vi "Parametrize.vi"(11 "Raw Data":dbl[][](array[numeric])) -> (3 "Poperties":T1)   [LabVIEW 2019]
uses:
  Communication/TypeDef/#TypeDef_PropertiesToSave.ctl
  Global_Freq.vi
  <vilib>/Analysis/NI_AALBase.lvlib
  <vilib>/Analysis/baseanly.llb/Mean (DBL).vi
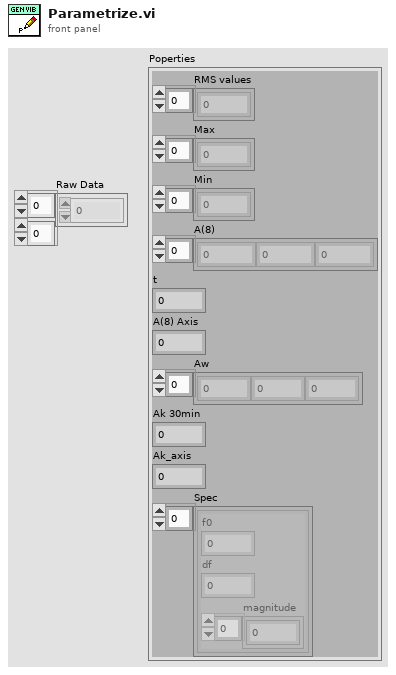
[diagram p1: front panel]
types:
  T1 = typedef "#TypeDef_PropertiesToSave.ctl" = cluster{"RMS values":dbl[], "Max":dbl[], "Min":dbl[], "A(8)":dbl[], "t":dbl, "A(8) Axis":dbl, "Aw":dbl[], "Ak 30min":dbl, "Ak_axis":i32, "Spec":cluster{"f0":dbl, "df":dbl, "magnitude":dbl[]}[]}
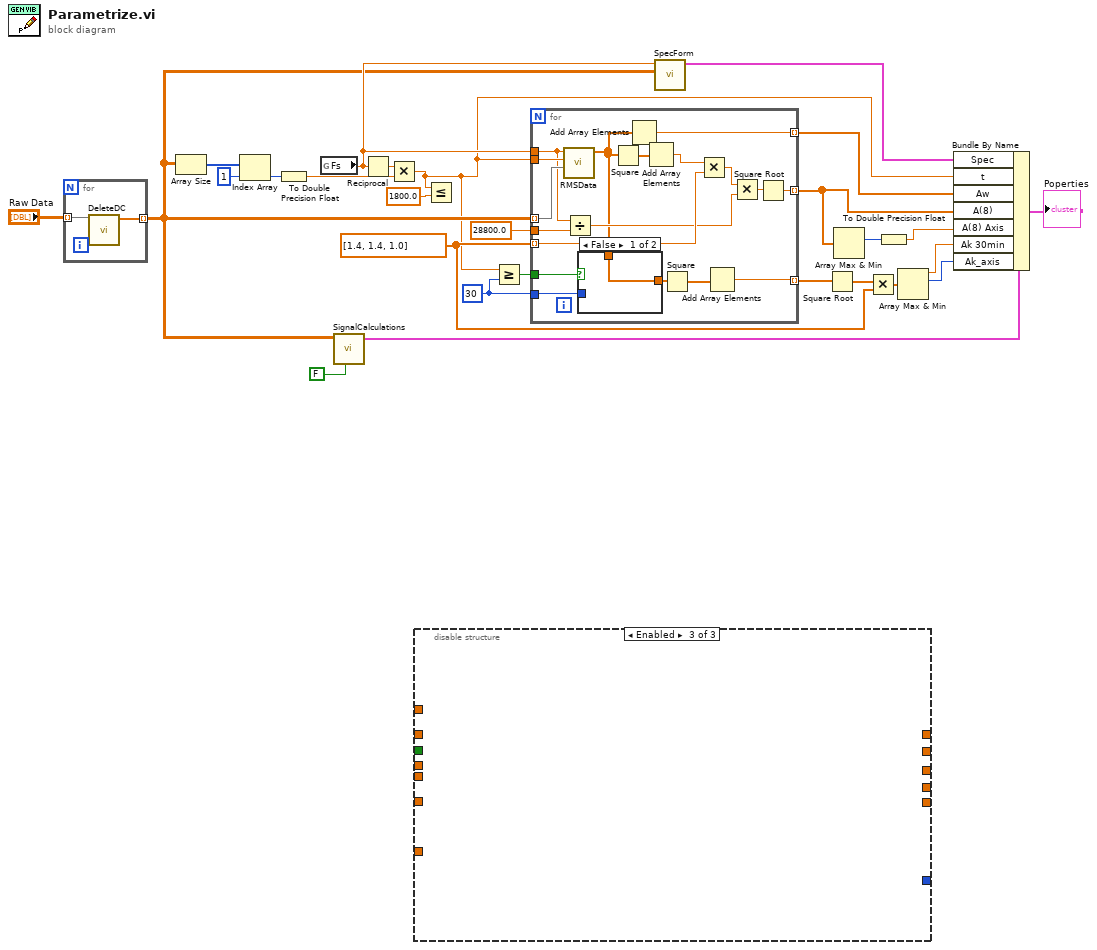
[diagram p0: block diagram]
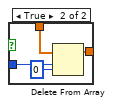
[diagram p2: hidden frame]
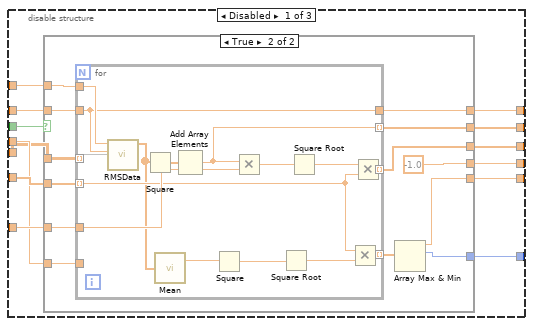
[diagram p3: hidden frame]
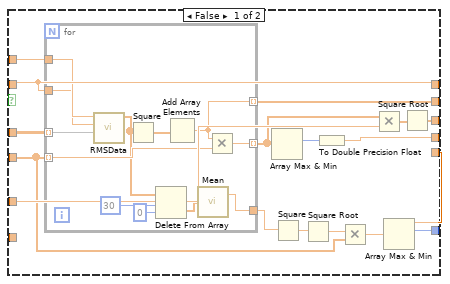
[diagram p4: hidden frame]
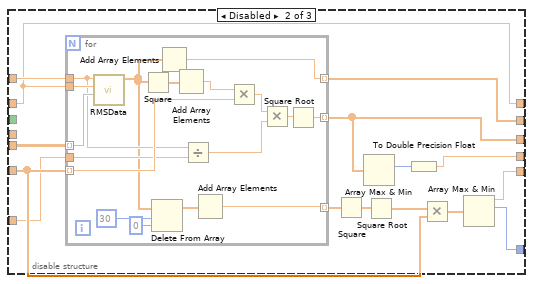
[diagram p5: hidden frame]
diagram:
  w3 = 30 ("length")
  w17 = dbl[] [1.4, 1.4, 1.0]
  n1 = for {
    tunnel: "Raw Data" -> [w29] mode=indexing
    tunnel: [w28] -> w8 mode=indexing
    n2 = call "DeleteDC.vi"("element"=w29) -> ("Array"=w28:dbl[])  [unwired: 10 in]
  }
  n3 = Array Size(array=w8) -> (size(s)=w18:i32[])
  n4 = Index Array(array=w18, index=1) -> (element=w20:i32)
  n5 = To Double Precision Float(number=w20) -> (double precision float=w14:dbl)
  n6 = global read "Global_Freq.vi" "Fs"() -> (w10:dbl)
  n7 = call "SignalCalculations.vi"("Ref?"=FALSE, "All Data"=w8) -> ("Poperties"=w23:T1)  [unwired: 8 in, 1 out]
  n8 = Reciprocal(x=w10) -> (1/x=w21:dbl)
  n9 = Multiply(x=w21, y=w14) -> (x*y=w2:dbl)
  n10 = disable-structure shown="Enabled" {
    disable-tunnel: [w42 w103 _] -> _
    disable-tunnel: [w41 w100 _] -> _
    disable-tunnel: [w40 w102 _] -> _
    disable-tunnel: [w39 w111 _] -> _
    disable-tunnel: _ -> [w38 w101 _]
    disable-tunnel: _ -> [w37 _ _]
    disable-tunnel: _ -> [w36 w111 _]
    disable-tunnel: _ -> [w35 w106 _]
    disable-tunnel: [w34 w105 _] -> _
    disable-tunnel: [w33 w104 _] -> _
    disable-tunnel: _ -> [w32 _ _]
    disable-tunnel: _ -> [w31 w112 _]
    disable-tunnel: _ -> [w30 w114 _]
    frame Disabled {
      n11 = case shown="True" w37 {
        tunnel: w35 -> [w43 w84]
        tunnel: [w57 w83] -> w41
        tunnel: w30 -> [w54 w82]
        tunnel: w36 -> [w44 w81]
        tunnel: w38 -> [w59 w80]
        tunnel: [w50 w79] -> w40
        tunnel: [w44 w78] -> w39
        tunnel: [w55 -1.0] -> w42
        tunnel: w32 -> [_ w76]
        tunnel: [w51 w74] -> w34
        tunnel: [w49 w73] -> w33
        tunnel: w31 -> [w45 w72]
        frame False {
          n12 = for {
            tunnel: w43 -> [w71] mode=indexing
            tunnel: w54 -> [w68] mode=indexing
            tunnel: [w70] -> w46 mode=indexing
            tunnel: [w66] -> w50 mode=indexing
            tunnel: [w60] -> w48
            tunnel: w45 -> [w64]
            tunnel: w44 -> [w63]
            n13 = call "RMSData.vi"("Data in"=w68, "t"=w63, "Fs"=w64) -> ("RMS Data out"=w62:dbl[])  [unwired: 8 in]
            n14 = Square(x=w62) -> (x^2=w67:dbl[])
            n15 = Delete From Array(array=w62, length=30, index=0) -> (deleted portion=w61:dbl[])  [unwired: 1 out]
            n16 = Add Array Elements(numeric array=w67) -> (sum=w66:dbl)
            n17 = call-poly <vilib>:"Mean.vi"("X"=w61) -> ("mean"=w60:dbl)  [unwired: 1 out]
            n18 = Multiply(x=w66, y=w71) -> (x*y=w70:dbl)
          }
          n19 = Array Max & Min(array=w46) -> (max index (indices)=w56:i32)  [unwired: 3 out]
          n20 = Square(x=w48) -> (x^2=w47:dbl)
          n21 = Square Root(x=w47) -> (sqrt(x)=w53:dbl)
          n22 = To Double Precision Float(number=w56) -> (double precision float=w55:dbl)
          n23 = Multiply(x=w53, y=w43) -> (x*y=w52:dbl)
          n24 = Multiply(x=w46, y=w59) -> (x*y=w58:dbl[])
          n25 = Array Max & Min(array=w52) -> (max value=w51:dbl, max index (indices)=w49:i32)  [unwired: 2 out]
          n26 = Square Root(x=w58) -> (sqrt(x)=w57:dbl[])
        }
        frame True {
          n27 = for {
            tunnel: w84 -> [w96] mode=indexing
            tunnel: [w99] -> w83 mode=indexing
            tunnel: w82 -> [w85] mode=indexing
            tunnel: w81 -> [w86]
            tunnel: w80 -> [w97]
            tunnel: [w92] -> w79 mode=indexing
            tunnel: [w86] -> w78
            tunnel: w76 -> [_]
            tunnel: [w95] -> w75 mode=indexing
            tunnel: w72 -> [w87]
            n28 = call "RMSData.vi"("Data in"=w85, "t"=w86, "Fs"=w87) -> ("RMS Data out"=w88:dbl[])  [unwired: 8 in]
            n29 = Square(x=w88) -> (x^2=w93:dbl[])
            n30 = call-poly <vilib>:"Mean.vi"("X"=w88) -> ("mean"=w89:dbl)  [unwired: 1 out]
            n31 = Add Array Elements(numeric array=w93) -> (sum=w92:dbl)
            n32 = Square(x=w89) -> (x^2=w91:dbl)
            n33 = Multiply(x=w92, y=w97) -> (x*y=w94:dbl)
            n34 = Square Root(x=w91) -> (sqrt(x)=w90:dbl)
            n35 = Square Root(x=w94) -> (sqrt(x)=w98:dbl)
            n36 = Multiply(x=w96, y=w90) -> (x*y=w95:dbl)
            n37 = Multiply(x=w98, y=w96) -> (x*y=w99:dbl)
          }
          n38 = Array Max & Min(array=w75) -> (max value=w74:dbl, max index (indices)=w73:i32)  [unwired: 2 out]
        }
      }
    }
    frame Disabled {
      n39 = for {
        tunnel: w106 -> [w131] mode=indexing
        tunnel: w114 -> [w127] mode=indexing
        tunnel: [w119] -> w100 mode=indexing
        tunnel: w112 -> [w124]
        tunnel: w111 -> [w128]
        tunnel: [w115] -> w102 mode=indexing
        tunnel: [w125] -> w107 mode=indexing
        tunnel: w101 -> [w123]
        n40 = call "RMSData.vi"("Data in"=w127, "t"=w128, "Fs"=w124) -> ("RMS Data out"=w116:dbl[])  [unwired: 8 in]
        n41 = Square(x=w116) -> (x^2=w118:dbl[])
        n42 = Delete From Array(array=w116, length=30, index=0) -> (array with subset deleted=w126:dbl[])  [unwired: 1 out]
        n43 = Add Array Elements(numeric array=w116) -> (sum=w115:dbl)
        n44 = Add Array Elements(numeric array=w118) -> (sum=w117:dbl)
        n45 = Divide(x=w124, y=w123) -> (x/y=w121:dbl)
        n46 = Add Array Elements(numeric array=w126) -> (sum=w125:dbl)
        n47 = Multiply(x=w117, y=w131) -> (x*y=w122:dbl)
        n48 = Multiply(x=w122, y=w121) -> (x*y=w120:dbl)
        n49 = Square Root(x=w120) -> (sqrt(x)=w119:dbl)
      }
      n50 = Square(x=w107) -> (x^2=w108:dbl[])
      n51 = Array Max & Min(array=w100) -> (max index (indices)=w113:i32)  [unwired: 3 out]
      n52 = Square Root(x=w108) -> (sqrt(x)=w110:dbl[])
      n53 = To Double Precision Float(number=w113) -> (double precision float=w103:dbl)
      n54 = Multiply(x=w110, y=w106) -> (x*y=w109:dbl[])
      n55 = Array Max & Min(array=w109) -> (max value=w105:dbl, max index (indices)=w104:i32)  [unwired: 2 out]
    }
    frame Enabled {
    }
  }
  n56 = Less Or Equal?(x=w2, y=1800.0) -> ()  [unwired: 1 out]
  n57 = Greater Or Equal?(x=w2, y=w3) -> (x >= y?=w1:bool)
  n58 = for {
    tunnel: w17 -> [w149] mode=indexing
    tunnel: w8 -> [w147] mode=indexing
    tunnel: [w140] -> w25 mode=indexing
    tunnel: w10 -> [w145]
    tunnel: w2 -> [w148]
    tunnel: [w136] -> w24 mode=indexing
    tunnel: [w146] -> w4 mode=indexing
    tunnel: 28800.0 -> [w144]
    tunnel: w3 -> [w133]
    tunnel: w1 -> [w132]
    n59 = call "RMSData.vi"("Data in"=w147, "t"=w148, "Fs"=w145) -> ("RMS Data out"=w137:dbl[])  [unwired: 8 in]
    n60 = Divide(x=w145, y=w144) -> (x/y=w142:dbl)
    n61 = case shown="False" w132 {
      tunnel: w137 -> [w150 w153]
      tunnel: [w150 w152] -> w135
      tunnel: w133 -> [_ w151]
      frame False {
      }
      frame True {
        n62 = Delete From Array(array=w153, length=w151, index=0) -> (array with subset deleted=w152:dbl[])  [unwired: 1 out]
      }
    }
    n63 = Square(x=w137) -> (x^2=w139:dbl[])
    n64 = Add Array Elements(numeric array=w137) -> (sum=w136:dbl)
    n65 = Add Array Elements(numeric array=w139) -> (sum=w138:dbl)
    n66 = Square(x=w135) -> (x^2=w134:dbl[])
    n67 = Multiply(x=w138, y=w149) -> (x*y=w143:dbl)
    n68 = Add Array Elements(numeric array=w134) -> (sum=w146:dbl)
    n69 = Multiply(x=w143, y=w142) -> (x*y=w141:dbl)
    n70 = Square Root(x=w141) -> (sqrt(x)=w140:dbl)
  }
  n71 = call "SpecForm.vi"("Data"=w8, "Fs"=w10) -> ("Power Spectrum / PSD"=w12:cluster{"f0":dbl, "df":dbl, "magnitude":dbl[]}[])  [unwired: 9 in]
  n72 = Square Root(x=w4) -> (sqrt(x)=w6:dbl[])
  n73 = Array Max & Min(array=w25) -> (max index (indices)=w7:i32)  [unwired: 3 out]
  n74 = Multiply(x=w6, y=w17) -> (x*y=w5:dbl[])
  n75 = To Double Precision Float(number=w7) -> (double precision float=w26:dbl)
  n76 = Array Max & Min(array=w5) -> (max value=w16:dbl, max index (indices)=w15:i32)  [unwired: 2 out]
  n77 = Bundle By Name(cluster=w23, "Spec"=w12, "t"=w2, "Aw"=w24, "A(8)"=w25, "A(8) Axis"=w26, "Ak 30min"=w16, "Ak_axis"=w15) -> (→"Poperties":T1)
